vi "SENS_CORR_CSET_DATA_A_B.vi"(0 "VISA IN":refnum<visa-resource-name>, 1 "Error Term,PortA,PortB":string, 2 "Param":string, 5 "error in":errorcluster, 7 "Channel":i32) -> (14 "VISA Out":refnum<visa-resource-name>, 19 "error out":errorcluster)   [LabVIEW 2018, in "PNA-X.lvlib"]
doc: "SENSe<cnum>:CORRection:CSET:DATA <eterm, portA, portB,>[<param>,] <block> \n(Read-Write) Read or Write a specific error term from/to the Cal Set currently attached to the \nspecified channel. (For Advanced Users). \nParameters \n<cnum> Any existing channel number. If unspecified, value is set to 1 \n<eterm, portA, \nportB> \nError Term, Port pair of the specified error term. \nAlthough not all error terms use two port numbers, two are required by the \nPNA in all cases. Each port number must be between 1 and the number of ports \non the PNA. \nEDIR - directivity \nportA: the port at which directivity is measured \nportB: Not used, but must be a valid PNA port number. \nESRM - source match \nportA: the port at which source match is measured \nportB: Not used, but must be a valid PNA port number. \n1691\n\nERFT - reflection tracking \nportA: the port at which reflection tracking is measured \nportB: Not used, but must be a valid PNA port number. \nELDM - load match \nportA: the port at which load match is measured \nportB: the source port. \nLoad match is measured with a cable connected between the measured port \n(portA) and the source port (portB). \nThe cal system requires that the complete matrix of loadmatch arrays be filled. \nIn most cases you can measure loadmatch once at a port, driven by any other \nport. Then use that data for all variations of the receive port. (The exception is \nthe 3-port PNA models, which requires the loadmatch-measured port to be \ndriven by every other port.) \nFor example: Measure the loadmatch at port2 while driving port1. Then upload \nthis same data to the following arrays: \nELDM,2,1,<data> \nELDM,2,3,<data> \nELDM,2,4,<data> \nETRT - transmission tracking \nportA: the receive port \nportB: the source port for this measurement \nEXTLK - crosstalk \nportA: the receive port \nportB: the source port for this measurement \nERSPT - response tracking. \nportA: Not used, but must be a valid PNA port number. \nportB: Not used, but must be a valid PNA port number. \n1692\n\nERSPI - response isolation. \nportA: Not used, but must be a valid PNA port number. \nportB: Not used, but must be a valid PNA port number. \n<param> <string> - required ONLY when Eterm is response tracking (ERSPT) or \nresponse isolation (ERSPI). Specify the S-parameter, ratio, or unratioed \nmeasurement for which the Eterm applies. \nLogical receiver notation is allowed. Ratioed measurements do not require \nsource port to be specified. \nA full 4-port calibration requires the following terms be uploaded: \nPORT B \n1 2 3 4 \nP\nO\nR\nT \nA \n1 \nEDIR,1,1 \nERFT,1,1 \nESRM,1,1 \nELDM,1,2 \nETRT,1,2 \nEXTLK,1,2 \nELDM,1,3 \nETRT,1,3 \nEXTLK,1,3 \nELDM,1,4 \nETRT,1,4 \nEXTLK,1,4 \n2 \nELDM,2,1 \nETRT,2,1 \nEXTLK,2,1 \nEDIR,2,2 \nERFT,2,2 \nESRM,2,2 \nELDM,2,3 \nETRT,2,3 \nEXTLK,2,3 \nELDM,2,4 \nETRT,2,4 \nEXTLK,2,4 \n3 \nELDM,3,1 \nETRT,3,1 \nEXTLK,3,1 \nELDM,3,2 \nETRT,3,2 \nEXTLK,3,2 \nEDIR,3,3 \nERFT,3,3 \nESRM,3,3 \nELDM,3,4 \nETRT,3,4 \nEXTLK,3,4 \n4 \nELDM,4,1 \nETRT,4,1 \nEXTLK,4,1 \nELDM,4,2 \nETRT,4,2 \nEXTLK,4,2 \nELDM,4,3 \nETRT,4,3 \nEXTLK,4,3 \nEDIR,4,4 \nERFT,4,4 \nESRM,4,4 \nReflection terms \nTransmission terms \nExamples SENS:CORR:CSET:DATA EXTLK,3,1 'cross talk between port 3 receiver \nand port 1 source. \nSENS:CORR:CSET:DATA ERSPT,1,1, \"a3/b4\" 'response tracking term \nfor ratioed measurement of port 4 test receiver over port 3 \nreference receiver. \n1693\n\nQuery Syntax SENSe<cnum>:CORRection:CSET:DATA? <eterm,portA, portB> \nReturn Type Block data \nDefault Not Applicable \nSENSe:CORRection:CSET:DELete <string> \n(Write-only) Deletes a Cal Set from the list of available Cal Sets. \nParameters \n<string> The GUID of the Cal Set to be deleted. The curly brackets and hyphens must \nbe included. Not case sensitive. \nExamples SENS:CORR:CSET:DEL '{2B893E7A-971A-11d5-8D6C-00108334AE96}' \nsense2:correction:cset:delete '{2B893E7A-971A-11d5-8D6C- \n00108334AE96}' \nQuery Syntax Not Applicable \nDefault Not Applicable"
uses:
  PNA-X.lvlib
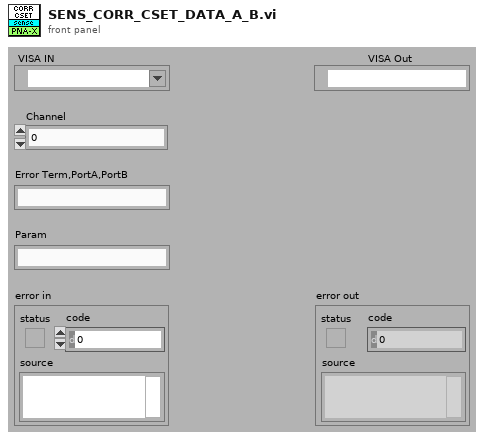
[diagram p1: front panel]
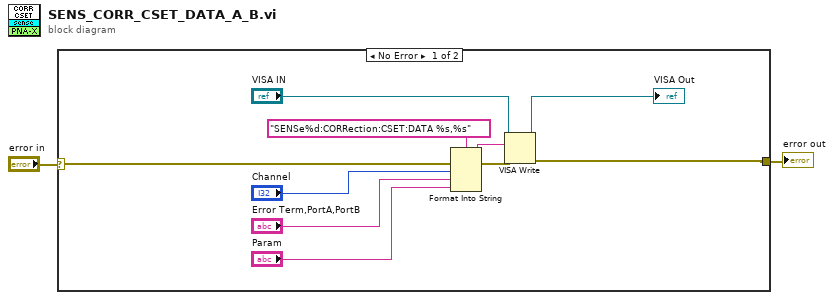
[diagram p0: block diagram]
diagram:
  n1 = case shown="No Error" "error in" {
    selector: "error in" -> [w12 w13]
    tunnel: [w7 w13] -> w1
    frame No Error {
      n2 = Format Into String(format string="SENSe%d:CORRection:CSET:DATA %s,%s" ("Cmdline"), error in=w12, "Channel", "Error Term,PortA,PortB", "Param") -> (resulting string=w10:string, error out=w11:errorcluster)  [unwired: 1 in]
      n3 = VISA Write(VISA resource name="VISA IN", write buffer=w10, error in (no error)=w11) -> (VISA resource name out=→"VISA Out":refnum<visa-resource-name>, error out=w7:errorcluster)  [unwired: 1 out]
    }
    frame Error {
    }
  }
  "error out" <- w1
